vi "BMark_User Visible Strings.vi"() -> ()   [LabVIEW 2016]
panel:
  in  "Switch App Instance":string="LabVIEW无法定位指定的应用程序实例。 " caption="切换应用程序实例"
  in  "Cannot Highlight (missing)":string="该标签的引用不再有效。" caption="无法高亮显示（丢失）"
  in  "Cannot Highlight (lock)":string="锁定VI中的前面板对象（或者无程序框图的VI）无法被高亮显示。" caption="无法高亮显示（锁定）"
  in  "Cannot Highlight (VI moved)":string="试图打开已移动/删除/重命名的VI。" caption="无法高亮显示（VI已移动）"
  in  "Cannot Highlight (pwd)":string="对于密码保护的VI，如密码不在缓存中，则无法高亮显示其中的标签。" caption="无法高亮显示（密码）"
  in  "Cannot Highlight (run)":string="无法在运行VI及其子VI中高亮显示标签。" caption="无法高亮显示（运行）"
  in  "Populating list":string="正在生成列表...请稍候" caption="生成列表"
  in  "More Information":string="更多信息" caption="更多信息"
  in  "no bookmarks found":string="未找到书签。" caption="未找到书签"
  in  "Bookmarks":string="书签" caption="书签"
  in  "VIs":string="VI" caption="VI"
  in  "Main application instance":string="主应用程序实例" caption="主应用程序实例"
  in  "unknown message error":string="消息处理循环接收到无效的消息字符串：%s。" caption="未知消息错误"
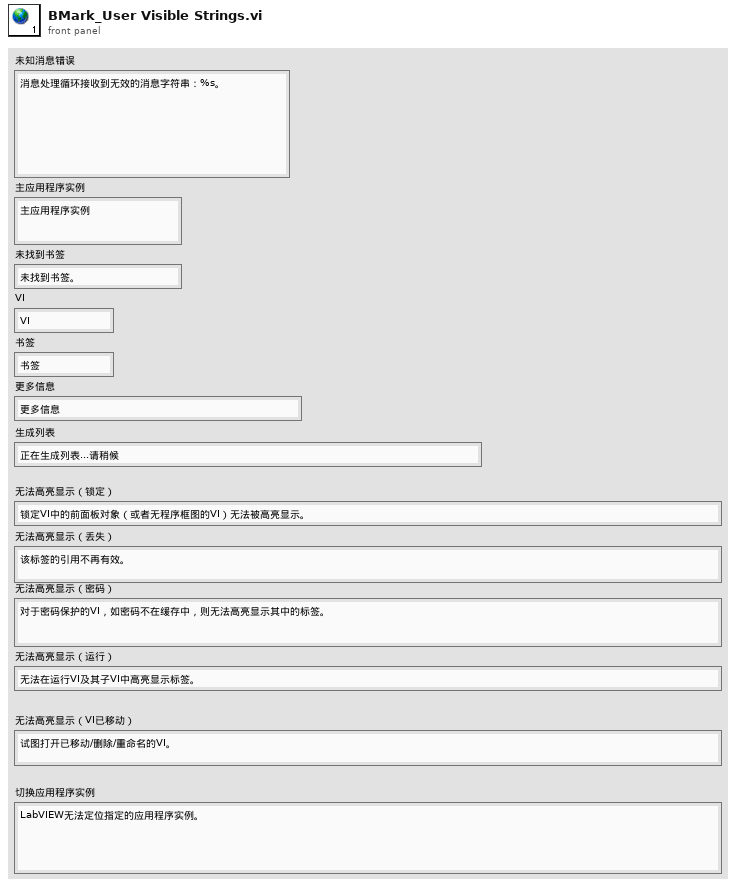
[diagram p1: front panel]
diagram:
